vi "Close Event FG.vi"(7 "Set (F)":bool, 11 "Close In":refnum<user-event>) -> (3 "Close":refnum<user-event>)   [LabVIEW 2020, in "Better Search.lvlib" / "BetterSearch.lvclass"]
uses:
  BetterSearch.lvclass
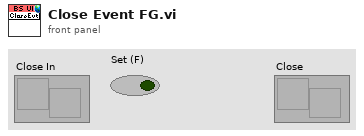
[diagram p1: front panel]
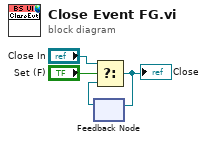
[diagram p0: block diagram]
diagram:
  n1 = feedback #1() -> (w2:refnum<user-event>)  [unwired: 1 in]
  n2 = Select(t="Close In", s="Set (F)", f=w2) -> (s? t:f=w1:refnum<user-event>)
  "Close" <- w1
  n3 = feedback-in #1(w1) -> ()
